vi "ADD TO LIST.vi"(8 "error in (no error)":errorcluster caption="错误输入（无错误）", 10 "List.lvlib:DATA.lvclass":refnum<class "DATA.lvclass">, 11 "List 输入":refnum<class "List.lvclass"> caption="DNL_LabVIEW Object in") -> (0 "error out":errorcluster caption="错误输出", 3 "List 输出":refnum<class "List.lvclass"> caption="DNL_LabVIEW Object out")   [LabVIEW 2011, in "List.lvlib" / "List.lvclass"]
uses:
  List.lvclass
  data/DATA.lvclass
  List.lvclass/List.ctl
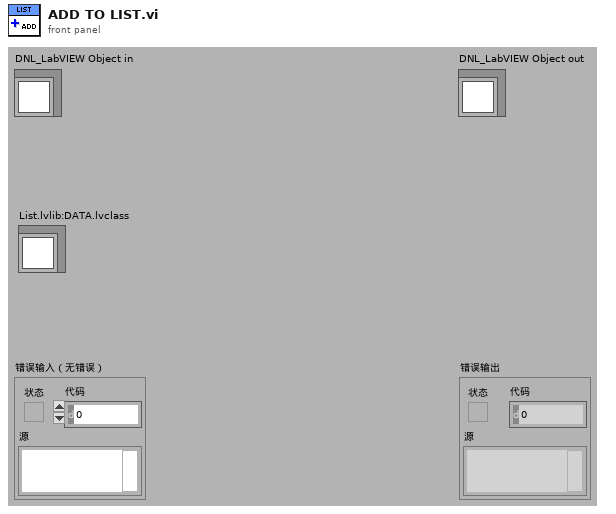
[diagram p1: front panel]
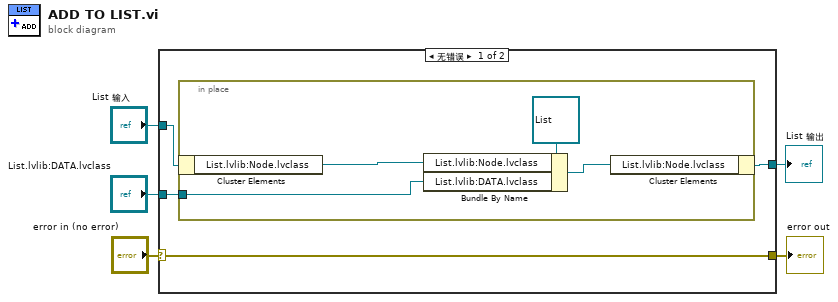
[diagram p0: block diagram]
diagram:
  n1 = case shown="无错误" "error in (no error)" {
    selector: "error in (no error)" -> [w9 w15]
    tunnel: [w9 w15] -> w4
    tunnel: [w7 w14] -> w2
    tunnel: "List 输入" -> [w8 w14]
    tunnel: "List.lvlib:DATA.lvclass" -> [w6 _]
    frame No Error {
      n2 = in-place {
        in-place-border: w6 -> [w12]
        n3 = in-place-cluster #1(w8) -> ("List.lvlib:Node.lvclass"=w11:refnum<class "Node.lvclass">)
        n4 = Bundle By Name(cluster=refnum<class "List.lvclass"> refnum ("List.lvlib:List.lvclass"), "List.lvlib:Node.lvclass"=w11, "List.lvlib:DATA.lvclass"=w12) -> (w10:refnum<class "List.lvclass">)
        n5 = in-place-cluster #1("List.lvlib:Node.lvclass"=w10) -> (w7:refnum<class "List.lvclass">)
      }
    }
    frame Error {
    }
  }
  "error out" <- w4
  "List 输出" <- w2
